vi "convert.vi"(10 "华氏?":bool, 11 "Data In in":T1 caption="Data In") -> (3 "Data In out":T1 caption="Data In")   [LabVIEW 2011, in "双模温度计.xctl"]
uses:
  Data.ctl
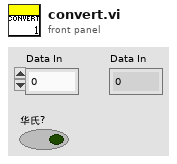
[diagram p1: front panel]
types:
  T1 = typedef "双模温度计.xctl/Data.ctl" = dbl
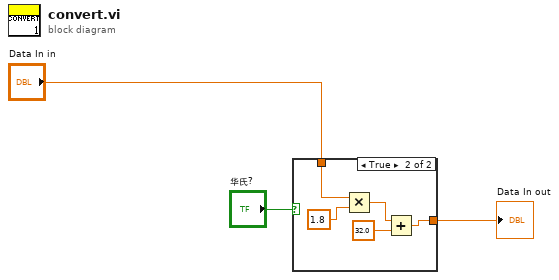
[diagram p0: block diagram]
diagram:
  n1 = case shown="True" "华氏?" {
    tunnel: "Data In in" -> [w4 w8]
    tunnel: [w4 w7] -> w3
    frame False {
    }
    frame True {
      n2 = Multiply(x=w8, y=T1 1.8) -> (x*y=w9:T1)
      n3 = Add(x=w9, y=T1 32.0) -> (x+y=w7:T1)
    }
  }
  "Data In out" <- w3
